vi "trim spaces.vi"(1 "multi-line string":string) -> (0 "result string":string)   [LabVIEW 2018]
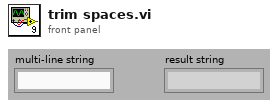
[diagram p1: front panel]
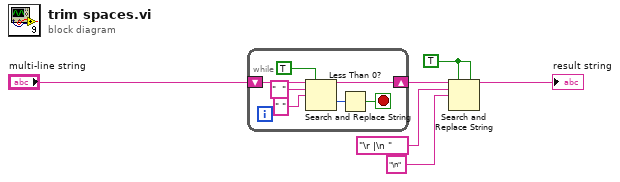
[diagram p0: block diagram]
diagram:
  w5 = TRUE ("replace all? (F)")
  n1 = while {
    shift-right: [w9] -> w3
    shift-left: "multi-line string" -> [w13]
    stop <- w7 stop-if-true
    n2 = Search and Replace String(replace all?=TRUE ("replace all? (F)"), input string=w13, search string="  ", replace string=" " ("search string")) -> (result string=w9:string, offset past replacement=w8:i32)  [unwired: 4 in, 2 out]
    n3 = Less Than 0?(x=w8) -> (x < 0?=w7:bool)
  }
  n4 = Search and Replace String(replace all?=w5, multiline?=w5, input string=w3, search string="\r |\n ", replace string="\n" ("search string")) -> (result string=→"result string":string)  [unwired: 3 in, 3 out]
